vi "systemid-hardware-recorder.vi"() -> ()   [LabVIEW 2012]
uses:
  <vilib>/rvi/interface/nirviMethod/nirviMethod.xnode
  <vilib>/rvi/interface/nirviReadWriteControl/nirviReadWriteControl.xnode
  <vilib>/Utility/file.llb/Write To Spreadsheet File (DBL).vi
  <vilib>/rvi/interface/nirviCloseFPGA/nirviCloseFPGA.xnode
  <vilib>/rvi/interface/nirviOpenFPGA/nirviOpenFPGA.xnode
  systemid-fpga-interface.vi
  <vilib>/rvi/errors/niLvFpgaMergeErrorWithErrorCode.vi
panel:
  out "sampleT":dbl
  out "decimate":i32 caption="Decimation Factor"
  out "Angle-FIFO Full":bool
  out "Voltage-FIFO Empty":bool
  out "Data File:":string
  out "Inputs":cluster{dbl[], dbl[]}(graph)
  out "Measurement":cluster{dbl[], dbl[]}(graph)
  out "DAQdone":bool
  in  "Abort":bool
  out "Data File (Full)":path
  out "Volts":dbl=5.304106305020111
  out "F (Hz)":dbl
  out "Inputs":i32(listbox)
  # "Set the desired inputs in the left MathScript node on the block diagram."
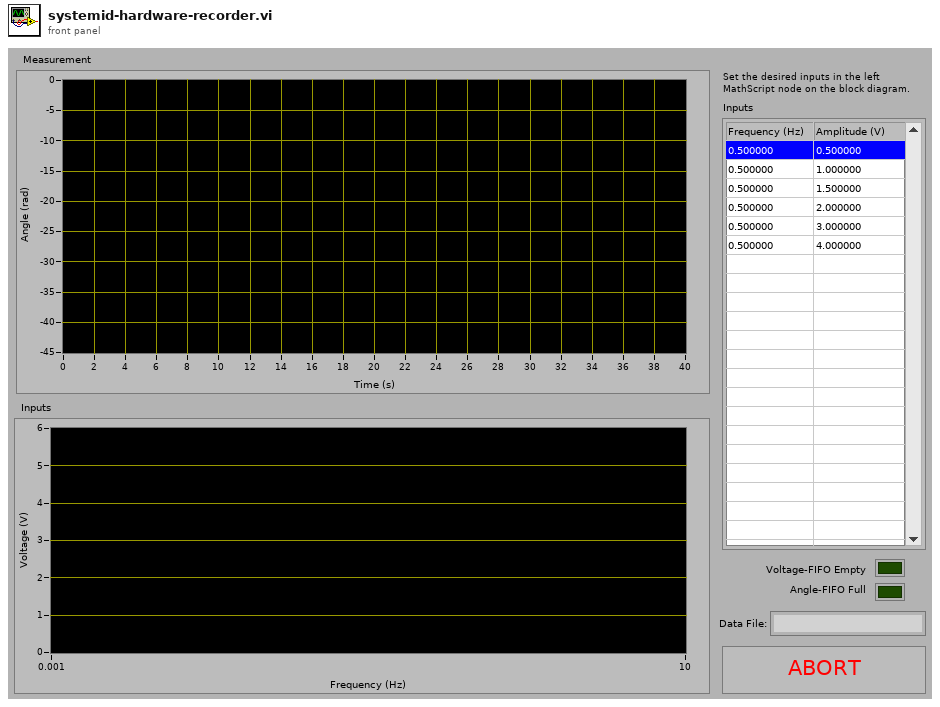
[diagram p1: front panel]
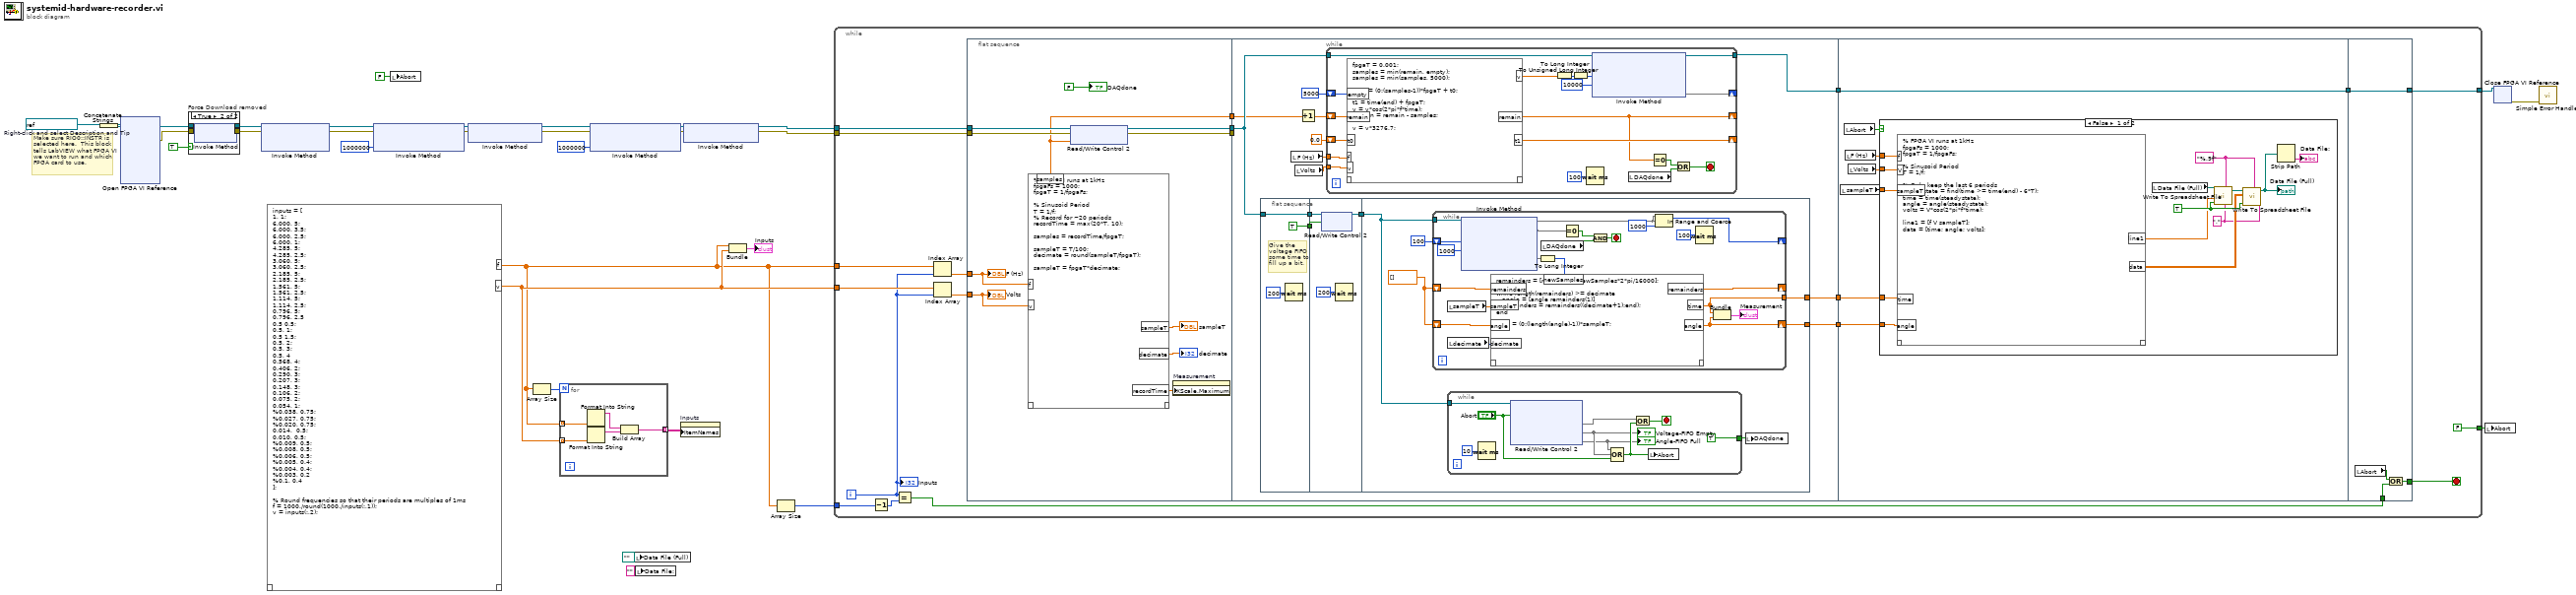
[diagram p0: block diagram]
diagram:
  # "Make sure RIO0::INSTR is selected here.  This block tells LabVIEW what FPGA VI we want to run and which FPGA card to use."
  n1 = Concatenate Strings "Right-click and select Description and Tip"(refnum<visa-resource-name> "RIO0::INSTR" ("resource name")) -> (w1:string)
  n2 = xnode "Open FPGA VI Reference"("resource name"=w1) -> ("FPGA VI Reference Out"=w27:refnum<k20>, "error out"=w20:errorcluster)  [unwired: 1 in]
  n3 = case "Force Download removed" shown="True" TRUE ("Force Download (F)") {
    tunnel: w27 -> [w33 w37]
    tunnel: [w33 w36] -> w13
    tunnel: w20 -> [w32 w35]
    tunnel: [w32 w34] -> w12
    frame False {
    }
    frame True {
      n4 = xnode "Invoke Method"("FPGA VI Reference In"=w37, "error in"=w35) -> ("FPGA VI Reference Out"=w36:refnum<k20>, "error out"=w34:errorcluster)
    }
  }
  n5 = xnode "Invoke Method"("FPGA VI Reference In"=w13, "error in"=w12) -> ("FPGA VI Reference Out"=w11:refnum<k20>, "error out"=w10:errorcluster)  [unwired: 1 in]
  n6 = mathscript code="inputs = [\n1, 1;\n6.000, 5;\n6.000, 3.5;\n6.000, 2.5;\n6.000, 1;\n4.285, 5;\n4.285, 2.5;\n3.060, 5;\n3.060, 2.5;\n2.185, 5; \n2.185, 2.5;\n1.561, 5;\n1.561, 2.5;\n1.114, 5;\n1.114, 2.5;\n0.796, 5;\n0.796, 2.5\n0.5 0.5;\n0.5, 1;\n0.5 1.5;\n0.5, 2;\n0.5, 3;\n0.5, 4\n0.568, 4;\n0.406, 2;\n0.290, 3;\n0.207, 3;\n0.148, 3;\n0.106, 2;\n0.075, 2;\n0.054, 1;\n%0.038, 0.75;\n%0.027, 0.75;\n%0.020, 0.75;\n0.014,  0.5;\n0.010, 0.5;\n%0.009, 0.5;\n%0.008, 0.5;\n%0.006, 0.5;\n%0.005, 0.4;\n%0.004, 0.4;\n%0.003, 0.2\n%0.1, 0.4\n];\n\n% Round frequencies so that their periods are multiples of 1ms\nf = 1000./round(1000./inputs(:,1));\nv = inputs(:,2);"() -> ("f"=w17:dbl[], "v"=w18:dbl[])  [unwired: 1 in, 1 out]
  n7 = xnode "Invoke Method"("FPGA VI Reference In"=w11, "error in"=w10, "Depth"=u32 1000000) -> ("FPGA VI Reference Out"=w9:refnum<k20>, "error out"=w8:errorcluster)
  n8 = local write "Abort"(FALSE ("Abort")) -> ()
  n9 = xnode "Invoke Method"("FPGA VI Reference In"=w9, "error in"=w8) -> ("FPGA VI Reference Out"=w7:refnum<k20>, "error out"=w4:errorcluster)
  n10 = Array Size(array=w17) -> (size(s)=w19:i32)
  n11 = for {
    N: w19 -> [_]
    tunnel: w17 -> [w42] mode=indexing
    tunnel: w18 -> [w41] mode=indexing
    tunnel: [w38] -> w16 mode=indexing
    n12 = Format Into String(w42) -> (resulting string=w40:string)  [unwired: 3 in, 1 out]
    n13 = Format Into String(w41) -> (resulting string=w39:string)  [unwired: 3 in, 1 out]
    n14 = Build Array(w40, w39) -> (w38:string[])
  }
  n15 = xnode "Invoke Method"("FPGA VI Reference In"=w7, "error in"=w4, "Depth"=u32 1000000) -> ("FPGA VI Reference Out"=w5:refnum<k20>, "error out"=w6:errorcluster)
  n16 = local write "Data File (Full)"(path "" ("Data File (Full)")) -> ()
  n17 = local write "Data File:"("" ("Data File:")) -> ()
  n18 = property on="Inputs" class="MCListbox (strict)"("ItemNames"=w16) -> ()  [unwired: 2 in, 2 out]
  n19 = xnode "Invoke Method"("FPGA VI Reference In"=w5, "error in"=w6) -> ("FPGA VI Reference Out"=w3:refnum<k20>, "error out"=w2:errorcluster)
  n20 = Bundle("f"=w17, "v"=w18) -> (→"Inputs":cluster{"f":dbl[], "v":dbl[]})  [unwired: 1 in]
  n21 = Array Size(array=w17) -> (size(s)=w28:i32)
  n22 = while {
    tunnel: w3 -> [w61]
    tunnel: [FALSE] -> w29
    tunnel: w28 -> [w48]
    tunnel: w17 -> [w59]
    tunnel: w18 -> [w57]
    tunnel: w2 -> [w55]
    tunnel: [w53] -> w15
    i -> [w47]
    stop <- w50 stop-if-true
    n23 = Decrement(x=w48) -> (x-1=w46:i32)
    n24 = Equal?(x=w47, y=w46) -> (x = y?=w49:bool)
    n25 = Index Array(array=w59, index=w47) -> (element=w58:dbl)
    n26 = Index Array(array=w57, index=w47) -> (element=w56:dbl)
    n27 = flat-sequence {
      tunnel: [w73] -> w62
      tunnel: w61 -> [w72]
      tunnel: w58 -> [w71]
      tunnel: w56 -> [w70]
      tunnel: w55 -> [w68]
      tunnel: [w67] -> w54
      tunnel: [w66] -> w44
      tunnel: w62 -> [w83]
      tunnel: w54 -> [_]
      tunnel: [w82] -> w52
      tunnel: [w81] -> w45
      tunnel: w44 -> [w74]
      tunnel: [w76] -> w43
      tunnel: w52 -> [w153]
      tunnel: [w153] -> w51
      tunnel: w45 -> [w147]
      tunnel: w43 -> [w149]
      tunnel: [w171] -> w53
      tunnel: w51 -> [w171]
      tunnel: [w170] -> w50
      tunnel: w49 -> [w168]
      frame #0 {
        n28 = mathscript code="% FPGA VI runs at 1kHz\nfpgaFs = 1000;\nfpgaT = 1/fpgaFs;\n\n% Sinusoid Period\nT = 1/f;\n% Record for ~20 periods\nrecordTime = max(20*T, 10);\n\nsamples = recordTime/fpgaT;\n\nsampleT = T/100;\ndecimate = round(sampleT/fpgaT);\n\nsampleT = fpgaT*decimate;"("f"=w71, "v"=w70) -> ("recordTime"=w65:dbl, "samples"=w66:dbl, "decimate"=→"decimate":dbl, "sampleT"=→"sampleT":dbl)  [unwired: 1 in, 1 out]
        n29 = xnode ("Read/Write Control 2")("FPGA VI Reference In"=w72, "error in"=w68, "Samples (1kHz)"=w66) -> ("FPGA VI Reference Out"=w73:refnum<k20>, "error out"=w67:errorcluster)
        n30 = property on="Measurement" class="XYGraph (strict)"("XScale.Maximum"=w65) -> ()  [unwired: 2 in, 2 out]
        "Volts" <- w70
        "F (Hz)" <- w71
        "DAQdone" <- FALSE ("DAQdone")
      }
      frame #1 {
        n31 = flat-sequence {
          tunnel: w83 -> [w88]
          tunnel: [w88] -> w84
          tunnel: [TRUE] -> w77
          tunnel: [w92] -> w85
          tunnel: w84 -> [w93]
          tunnel: w77 -> [w90]
          tunnel: w85 -> [w96]
          tunnel: [w95] -> w81
          tunnel: [w94] -> w76
          frame #0 {
            # "Give the voltage FIFO some time to fill up a bit."
            n32 = Wait (ms)(milliseconds to wait=u32 200) -> ()  [unwired: 1 out]
          }
          frame #1 {
            n33 = xnode ("Read/Write Control 2")("FPGA VI Reference In"=w93, "Start"=w90) -> ("FPGA VI Reference Out"=w92:refnum<k20>)  [unwired: 1 in, 1 out]
            n34 = Wait (ms)(milliseconds to wait=u32 200) -> ()  [unwired: 1 out]
          }
          frame #2 {
            w97 = dbl[] [] ("first subarray")
            n35 = while {
              shift-right: [w118] -> _
              shift-left: u32 100 -> [w117]
              shift-right: [w108] -> _
              shift-left: w97 -> [w106]
              tunnel: w96 -> [w119]
              shift-right: [w103] -> w95
              shift-left: w97 -> [w107]
              tunnel: [w101] -> w94
              stop <- w112 stop-if-true
              n36 = local read "sampleT"() -> (w105:dbl)
              n37 = local read "decimate"() -> (w100:i32)
              n38 = xnode "Invoke Method"("FPGA VI Reference In"=w119, "Number of Elements"=w117, "Timeout (ms)"=1000) -> ("Data"=w115:void[], "Elements Remaining"=w113)  [unwired: 1 in, 2 out]
              n39 = To Long Integer(number=w115) -> (32bit integer=w104:i32[])
              n40 = mathscript code="remainders = [remainders newSamples*2*pi/16000];\n\nwhile length(remainders) >= decimate\n   angle = [angle remainders(1)]\n   remainders = remainders((decimate+1):end);\nend\n\ntime = (0:(length(angle)-1))*sampleT;"("newSamples"=w104, "remainders"=w106, "angle"=w107, "sampleT"=w105, "decimate"=w100) -> ("remainders"=w108:dbl[], "time"=w101:dbl[], "angle"=w103:dbl[])  [unwired: 1 in, 1 out]
              n41 = local read "DAQdone"() -> (w111:bool)
              n42 = Equal To 0?(x=w113) -> (x = 0?=w110:bool)
              n43 = And(x=w110, y=w111) -> (x .and. y?=w112:bool)
              n44 = In Range and Coerce(upper limit=w113, x=w113, lower limit=u32 1000) -> (coerced(x)=w118:u32)  [unwired: 1 out]
              n45 = Wait (ms)(milliseconds to wait=u32 100) -> ()  [unwired: 1 out]
              n46 = Bundle("time"=w101, "angle"=w103) -> (→"Measurement":cluster{"time":dbl[], "angle":dbl[]})  [unwired: 1 in]
            }
            n47 = while {
              tunnel: [TRUE ("DAQdone")] -> w99
              tunnel: w96 -> [w125]
              stop <- w127 stop-if-true
              n48 = Wait (ms)(milliseconds to wait=u32 10) -> ()  [unwired: 1 out]
              n49 = xnode ("Read/Write Control 2")("FPGA VI Reference In"=w125, "Abort"="Abort") -> ("Idle"=w124, "Voltage-In-Empty"=w121, "Angle-Out-FIFO Full"=w120)  [unwired: 1 in, 2 out]
              "Voltage-FIFO Empty" <- w121
              "Angle-FIFO Full" <- w120
              n50 = Compound Arithmetic op=OR(w120, w121, "Abort") -> (w122:bool)
              n51 = Or(x=w124, y=w122) -> (x .or. y?=w127:bool)
              n52 = local write "Abort"(w122) -> ()
            }
            n53 = local write "DAQdone"(w99) -> ()
          }
        }
        n54 = local read "F (Hz)"() -> (w79:dbl)
        n55 = local read "Volts"() -> (w78:dbl)
        n56 = Increment(x=w74) -> (x+1=w75:dbl)
        n57 = while {
          shift-right: [w140] -> _
          shift-left: 5000 -> [w136]
          tunnel: w83 -> [w144]
          tunnel: [w141] -> w82
          shift-right: [w138] -> _
          shift-left: 0.0 -> [w137]
          tunnel: w79 -> [w135]
          tunnel: w78 -> [w134]
          shift-right: [w130] -> _
          shift-left: w75 -> [w132]
          stop <- w146 stop-if-true
          n58 = mathscript code="fpgaT = 0.001;\nsamples = min(remain, empty);\nsamples = min(samples, 5000);\n\ntime = (0:(samples-1))*fpgaT + t0;\n\nt1 = time(end) + fpgaT;\nv = v*cos(2*pi*f*time);\nremain = remain - samples;\n\nv = v*3276.7;"("f"=w135, "v"=w134, "t0"=w137, "empty"=w136, "remain"=w132) -> ("v"=w129:dbl[], "t1"=w138:dbl, "remain"=w130:dbl)  [unwired: 1 in, 1 out]
          n59 = To Long Integer(number=w129) -> (32bit integer=w142:i32[])
          n60 = To Unsigned Long Integer(number=w142) -> (unsigned 32bit integer=w139:u32[])
          n61 = Wait (ms)(milliseconds to wait=u32 100) -> ()  [unwired: 1 out]
          n62 = xnode "Invoke Method"("FPGA VI Reference In"=w144, "Data"=w139, "Timeout (ms)"=10000) -> ("FPGA VI Reference Out"=w141:refnum<k20>, "Empty Elements Remaining"=w140)  [unwired: 1 in, 1 out]
          n63 = local read "DAQdone"() -> (w145:bool)
          n64 = Equal To 0?(x=w130) -> (x = 0?=w131:bool)
          n65 = Or(x=w131, y=w145) -> (x .or. y?=w146:bool)
        }
      }
      frame #2 {
        n66 = local read "sampleT"() -> (w148:dbl)
        n67 = local read "Abort"() -> (w152:bool)
        n68 = local read "F (Hz)"() -> (w151:dbl)
        n69 = local read "Volts"() -> (w150:dbl)
        n70 = case shown="False" w152 {
          tunnel: w150 -> [w161 _]
          tunnel: w151 -> [w160 _]
          tunnel: w147 -> [w157 _]
          tunnel: w149 -> [w156 _]
          tunnel: w148 -> [w155 _]
          frame False {
            w154 = "," ("delimiter (\\t)")
            w165 = TRUE ("append to file? (new file:F)")
            w166 = "%.9f" ("format (%.3f)")
            n71 = mathscript code="% FPGA VI runs at 1kHz\nfpgaFs = 1000;\nfpgaT = 1/fpgaFs;\n\n% Sinusoid Period\nT = 1/f;\n\n% Only keep the last 6 periods\nsteadystate = find(time >= time(end) - 6*T);\ntime = time(steadystate);\nangle = angle(steadystate);\nvolts = V*cos(2*pi*f*time);\n\nline1 = [f V sampleT];\ndata = [time; angle; volts];"("f"=w160, "V"=w161, "time"=w156, "angle"=w157, "sampleT"=w155) -> ("line1"=w159:dbl[], "data"=w158:dbl[][])  [unwired: 1 in, 1 out]
            n72 = local read "Data File (Full)"() -> (w164:path)
            n73 = call-poly <vilib>:"Write To Spreadsheet File.vi"("delimiter (\\t)"=w154, "format (%.3f)"=w166, "append to file? (new file:F)"=w165, "1D data"=w159, "file path (dialog if empty)"=w164) -> ("new file path (Not A Path if cancelled)"=w167:path)  [unwired: 3 in]
            n74 = call-poly <vilib>:"Write To Spreadsheet File.vi"("delimiter (\\t)"=w154, "format (%.3f)"=w166, "append to file? (new file:F)"=w165, "2D data"=w158, "file path (dialog if empty)"=w167) -> ("new file path (Not A Path if cancelled)"=w163:path)  [unwired: 3 in]
            "Data File (Full)" <- w163
            n75 = Strip Path(path=w163) -> (name=→"Data File:":string)  [unwired: 1 out]
          }
          frame True {
          }
        }
      }
      frame #3 {
        n76 = local read "Abort"() -> (w169:bool)
        n77 = Or(x=w169, y=w168) -> (x .or. y?=w170:bool)
      }
    }
    "Inputs" <- w47
  }
  n78 = local write "Abort"(w29) -> ()
  n79 = xnode "Close FPGA VI Reference"("FPGA VI Reference In"=w15) -> ("error out"=w30:errorcluster)  [unwired: 1 in]
  n80 = call <vilib>:"Simple Error Handler.vi"("error in (no error)"=w30) -> ()  [unwired: 4 in, 5 out]
